vi "Any2DBoolean.vi"(8 "Dimension (0)":u16, 11 "2D Boolean Array":bool[][](array[boolean])=[[FALSE, FALSE, FALSE, FALSE, FALSE], [FALSE, FALSE, FALSE, FALSE, FALSE], [FALSE, FALSE, FALSE, FALSE, FALSE]]) -> (3 "1D Array":bool[](array[boolean]))   [LabVIEW 2016]
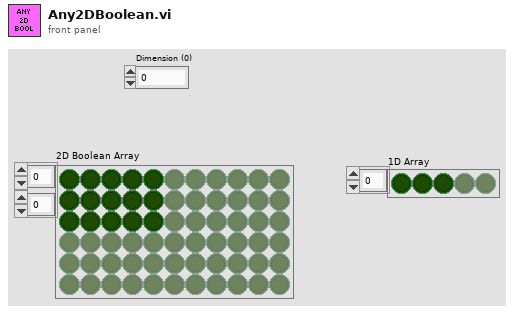
[diagram p1: front panel]
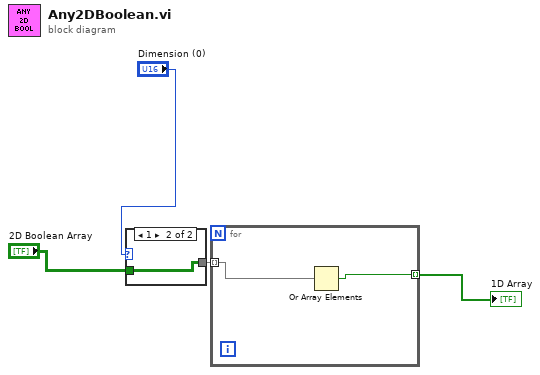
[diagram p0: block diagram]
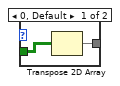
[diagram p2: hidden frame]
diagram:
  n1 = case shown="1" "Dimension (0)" {
    tunnel: "2D Boolean Array" -> [w6 w7]
    tunnel: [w5 w7] -> w2
    frame 0, Default {
      n2 = Transpose 2D Array(2D array=w6) -> (transposed array=w5:bool[][])
    }
    frame 1 {
    }
  }
  n3 = for {
    tunnel: w2 -> [w9] mode=indexing
    tunnel: [w8] -> w1 mode=indexing
    n4 = Or Array Elements(Boolean array=w9) -> (logical OR=w8:bool)
  }
  "1D Array" <- w1
